vi "Set Name Value Pairs.vi"(8 "error in (no error)":errorcluster, 9 "Object (or Item) Path":string, 10 "Properties":T1[](array[typedef]), 11 "CycloneDX JSON in":refnum<class "CycloneDX JSON.lvclass">) -> (0 "error out":errorcluster, 3 "CycloneDX JSON out":refnum<class "CycloneDX JSON.lvclass">)   [LabVIEW 2017, in "LabVIEW CycloneDX SBOM.lvlib" / "CycloneDX JSON.lvclass"]
uses:
  CycloneDX JSON.lvclass
  Name Value Pair.ctl
  b6ee377a-5e63-4960-ae3c-195e2d7e4347.vi
  <vilib>/JDP Science/JSONtext/Variant to JSON Text.vi
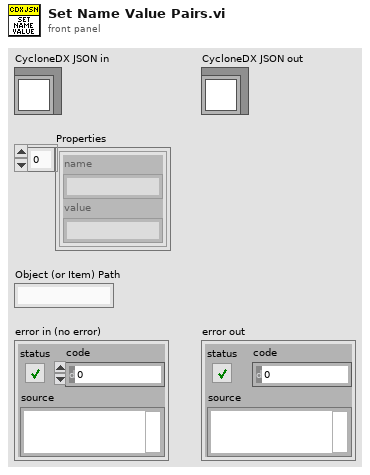
[diagram p1: front panel]
types:
  T1 = typedef "LabVIEW CycloneDX SBOM.lvlib/CycloneDX JSON.lvclass/Name Value Pair.ctl" = cluster{"name":string, "value":string}
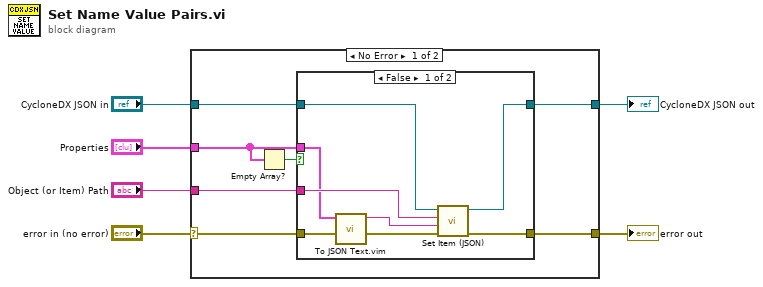
[diagram p0: block diagram]
diagram:
  n1 = case shown="No Error" "error in (no error)" {
    selector: "error in (no error)" -> [w10 w25]
    tunnel: "Properties" -> [w12 _]
    tunnel: [w11 w25] -> w5
    tunnel: [w9 w24] -> w3
    tunnel: "CycloneDX JSON in" -> [w8 w24]
    tunnel: "Object (or Item) Path" -> [w7 _]
    frame No Error {
      n2 = Empty Array?(array=w12) -> (empty?=w13:bool)
      n3 = case shown="False" w13 {
        tunnel: w7 -> [w21 _]
        tunnel: w8 -> [w20 w23]
        tunnel: [w19 w23] -> w9
        tunnel: w10 -> [w15 w22]
        tunnel: [w18 w22] -> w11
        tunnel: w12 -> [w16 _]
        frame False {
          n4 = call "To JSON Text.vim"("error in (no error)"=w15, "Anything"=w16) -> ("error out"=w14:errorcluster, "<JSON>"=w17:string)  [unwired: 8 in]
          n5 = call "Set Item (JSON).vi"("error in (no error)"=w14, "JSON to Insert"=w17, "Object (or Item) Path"=w21, "CycloneDX SBOM in"=w20) -> ("error out"=w18:errorcluster, "CycloneDX SBOM out"=w19:refnum<class "CycloneDX JSON.lvclass">)  [unwired: 6 in]
        }
        frame True {
        }
      }
    }
    frame Error {
    }
  }
  "error out" <- w5
  "CycloneDX JSON out" <- w3
